vi "test1-LocalExternalStatusRegistration.vi"(8 "error in (no error)":errorcluster, 11 "TestCase in":refnum<class "testcase-CSMBroadcast.lvclass">) -> (0 "error out":errorcluster, 3 "TestCase out":refnum<class "testcase-CSMBroadcast.lvclass">)   [LabVIEW 2017, in "testcase-CSMBroadcast.lvclass"]
uses:
  testcase-CSMBroadcast.lvclass
  0b17d103-e67b-41be-a9eb-a2ee1311ff1f.vi
  5999693e-4f8a-4b34-ae87-f34dff5771be.vi
  de2dcf32-e0f3-4ce3-ae15-c78c2a65fbc0.vi
  52a2a10a-a04b-4bad-8df4-e1eb944f47cc.vi
  826f03dd-b4b5-4c6b-9085-8edf6da4f43b.vi
  src/user.lib/_NEVSTOP/Communicable State Machine(CSM)/AdvanceAPI/CSM - Revert Arguments-Safe String.vi
  src/user.lib/_NEVSTOP/Communicable State Machine(CSM)/AdvanceAPI/CSM - Make String Arguments Safe.vi
  src/user.lib/_NEVSTOP/Communicable State Machine(CSM)/AdvanceAPI/CSM - Break Down Multiple States String.vi
  src/user.lib/_NEVSTOP/Communicable State Machine(CSM)/AdvanceAPI/CSM - Keywords.vi
  src/user.lib/_NEVSTOP/Communicable State Machine(CSM)/_Polymophic/CSM - Replace Marks in Messages.vi
  src/user.lib/_NEVSTOP/Communicable State Machine(CSM)/AdvanceAPI/CSM - Get Module Attribute.vi
  src/user.lib/_NEVSTOP/Communicable State Machine(CSM)/_Shared/Trim Single-line Text.vi
  <vilib>/addons/_JKI Toolkits/VI Tester/TestCase.llb/TestCase.lvclass
  src/user.lib/_NEVSTOP/Communicable State Machine(CSM)/Communicable State Machine.lvlib
  CSM/CSM-Testcase.lvlib
  C:/Program Files (x86)/National Instruments/LabVIEW 2017/vi.lib/addons/_JKI Toolkits/VI Tester/TestCase.llb/TestCase.lvclass
panel:
  out "One-Shot Unregistrations":string
  out "One-Shot Registrations":string
  out "LoopCount 2":i32
  out "State History":string
  out "LoopCount":i32
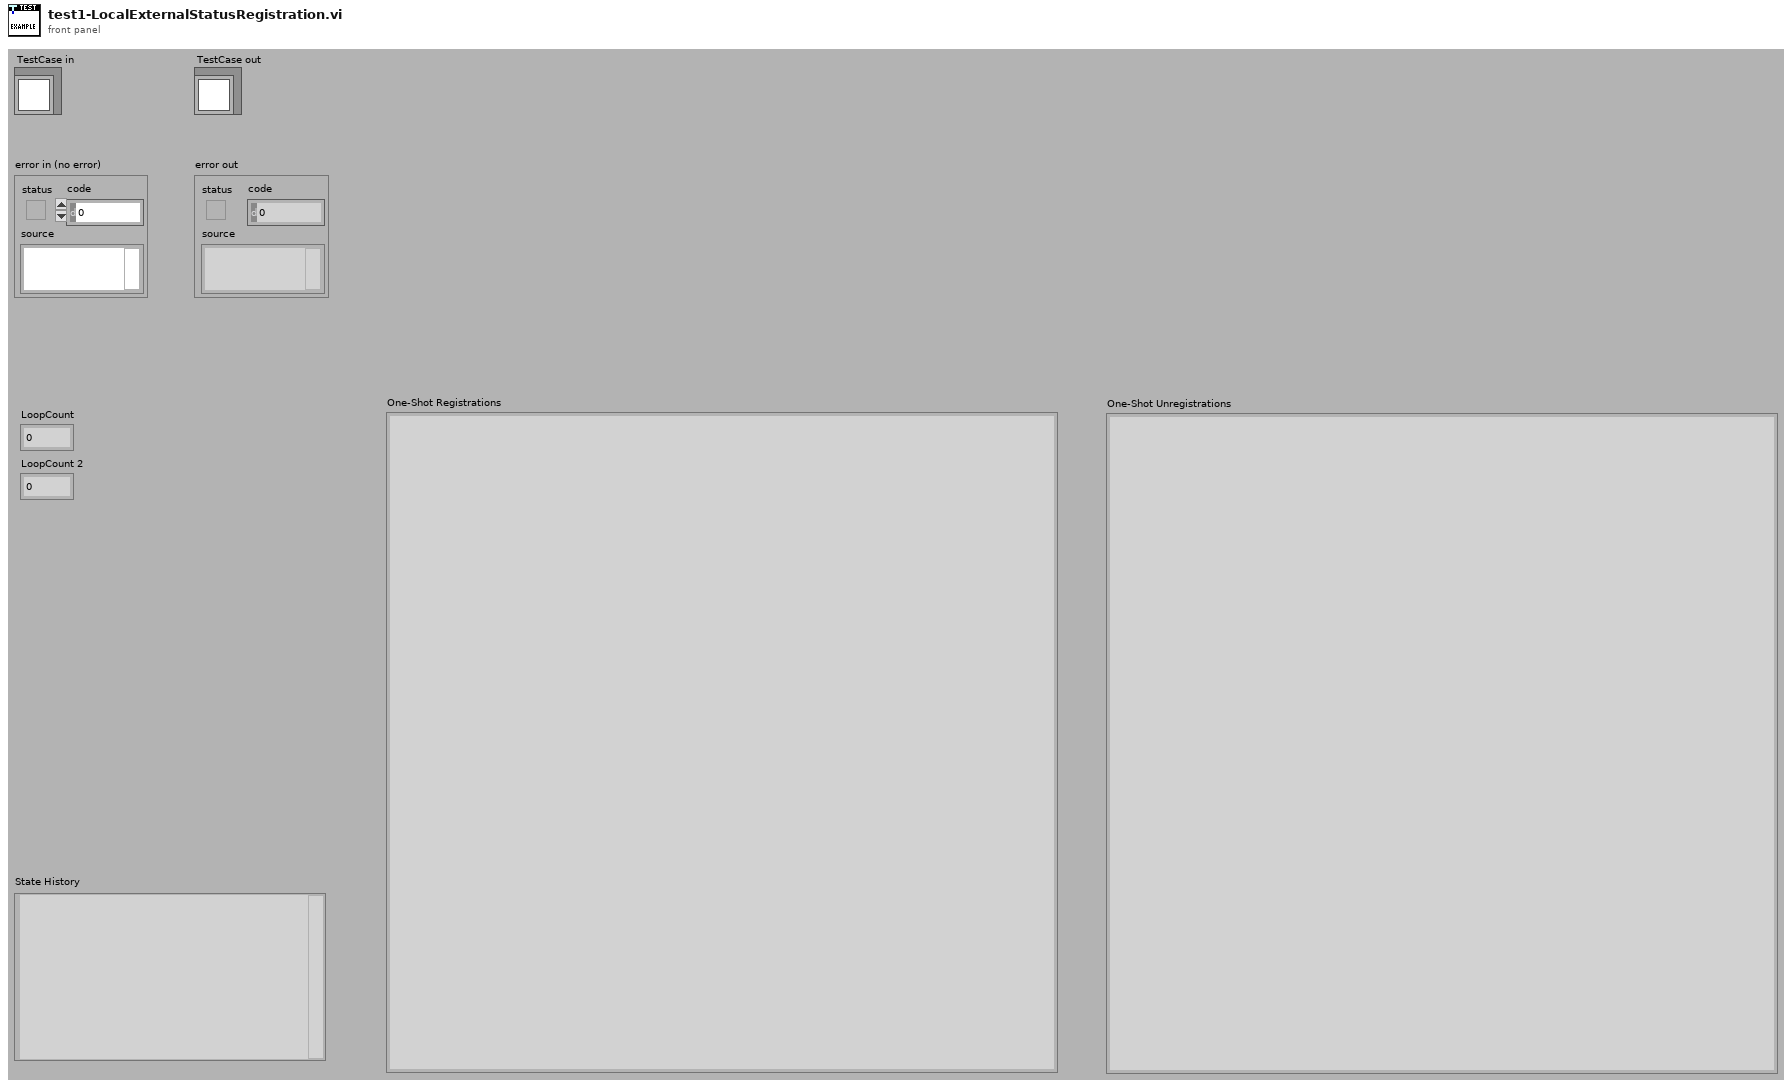
[diagram p1: front panel]
types:
  T1 = enum32{"Invalid", "Standard", "Closed", "Hidden", "Minimized", "Maximized"}
  T2 = enum32{"invalid app kind", "Development System", "Run Time System", "Student Edition", "Embedded LabVIEW", "Evaluation", "Custom"}
  T3 = typedef "Communicable State Machine.lvlib/_CSM_Response Source Message.ctl" = cluster{"‘State":string, "’Arguments":string, "’Error":errorcluster}
  T4 = cluster{"Current VI Reference":refnum<vi>, "Close Panel on Exit?":bool}
  T5 = cluster{"Core":cluster{"Current VI Reference":refnum<vi>, "Close Panel on Exit?":bool}, "Your Boolean data":bool, "Your string data":string}
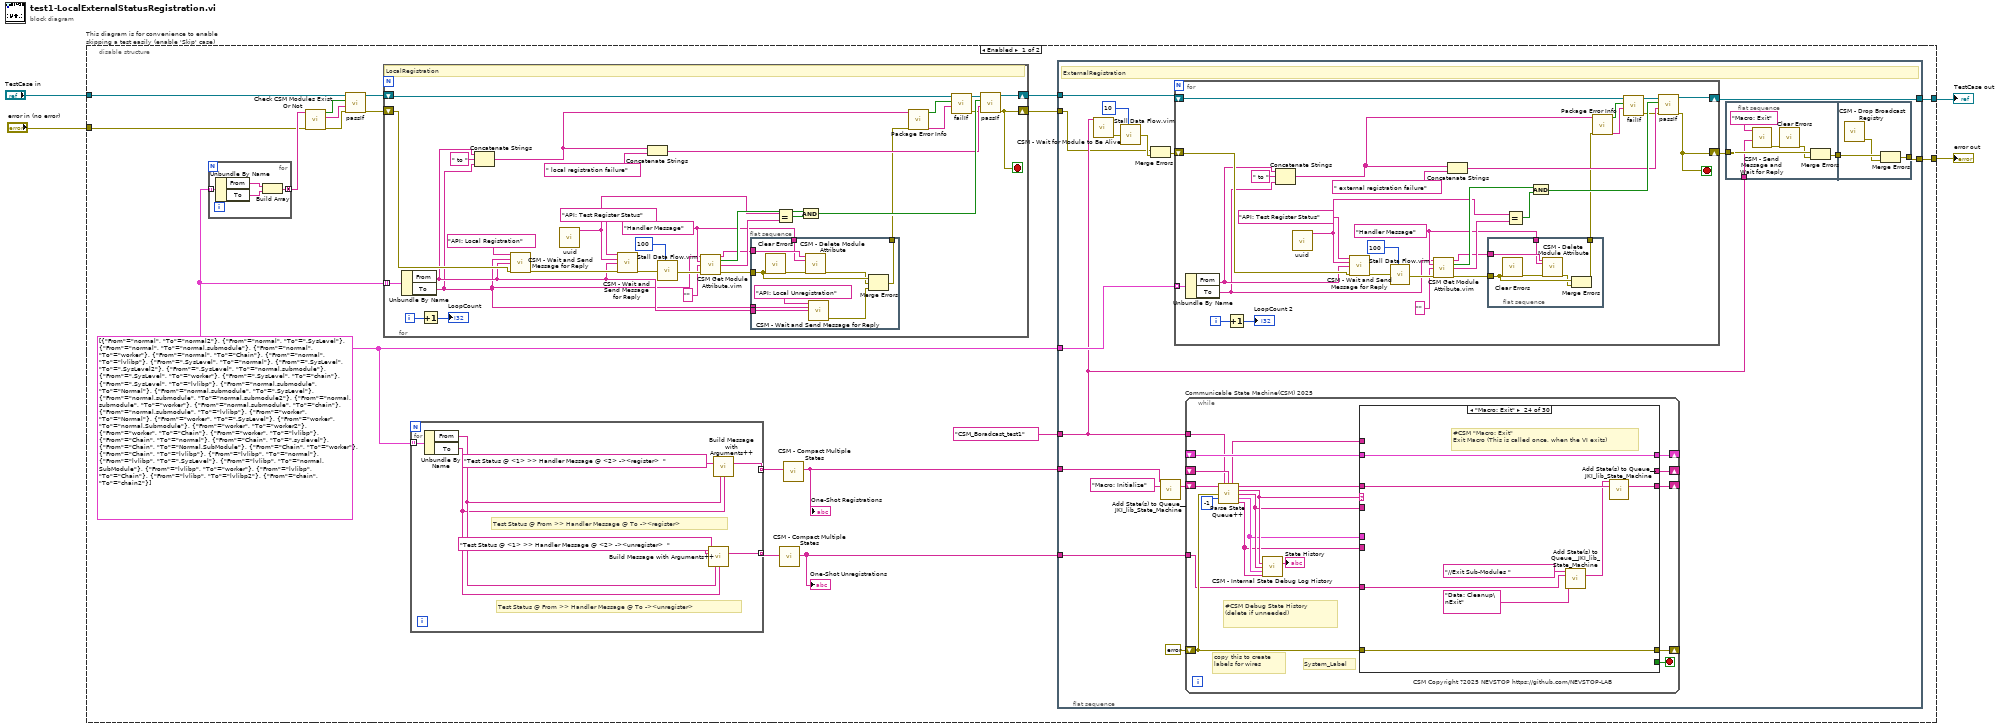
[diagram p0: block diagram]
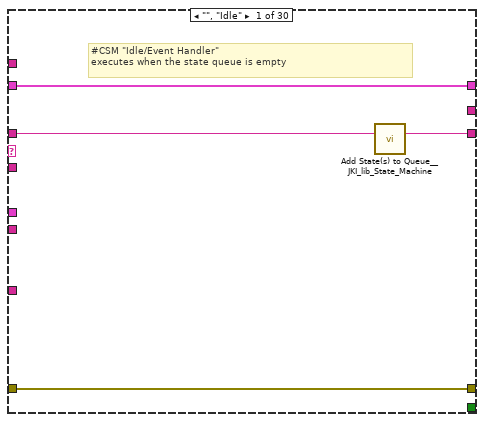
[diagram p2: hidden frame]
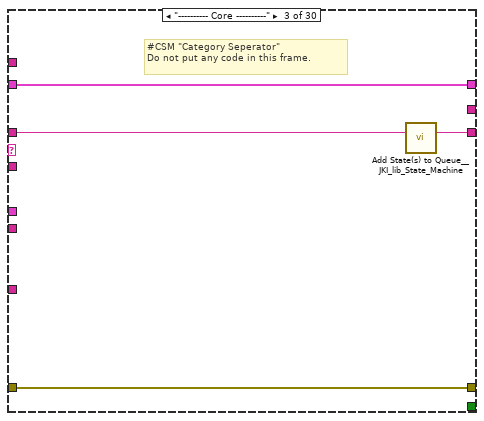
[diagram p4: hidden frame]
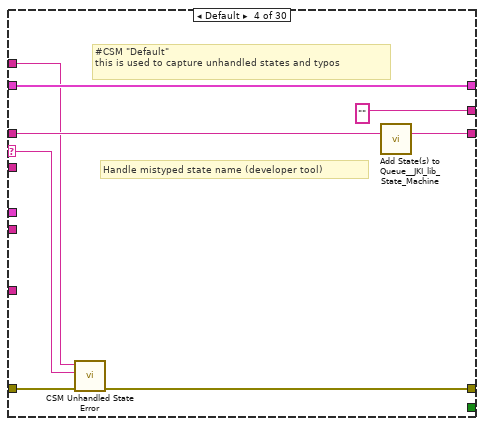
[diagram p5: hidden frame]
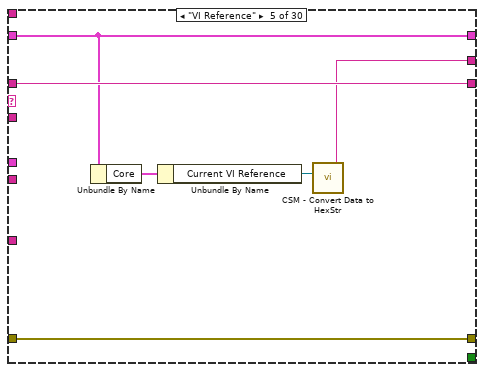
[diagram p6: hidden frame]
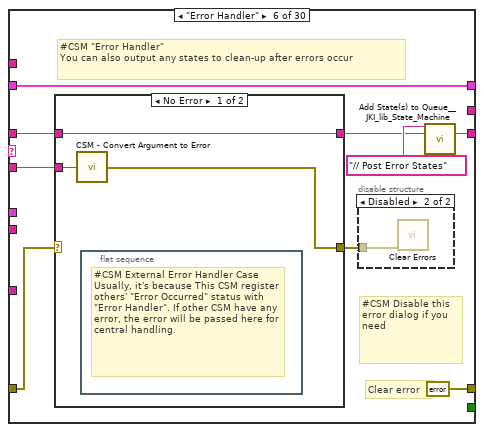
[diagram p7: hidden frame]
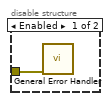
[diagram p8: hidden frame]
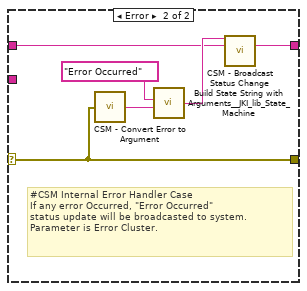
[diagram p9: hidden frame]
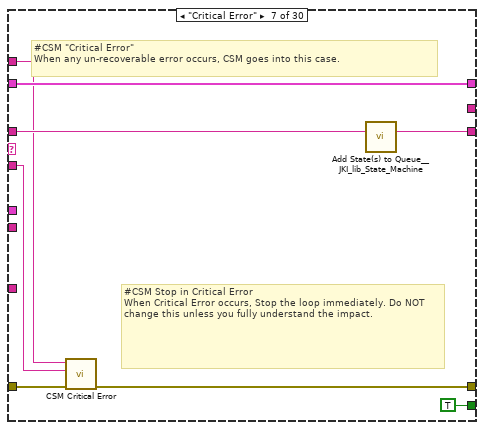
[diagram p10: hidden frame]
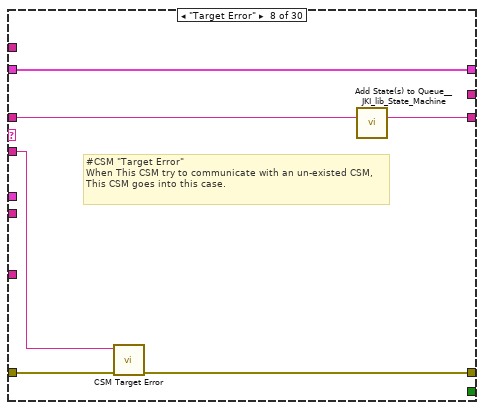
[diagram p11: hidden frame]
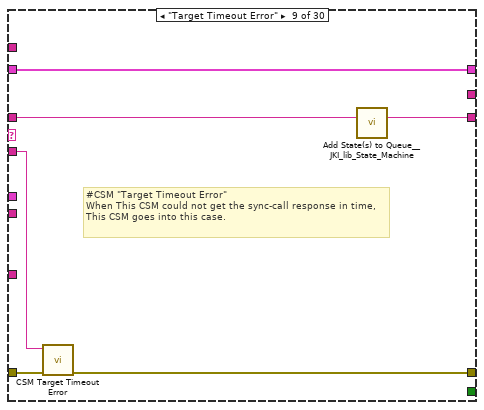
[diagram p12: hidden frame]
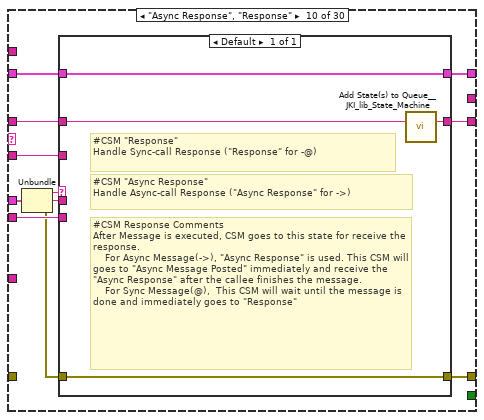
[diagram p13: hidden frame]
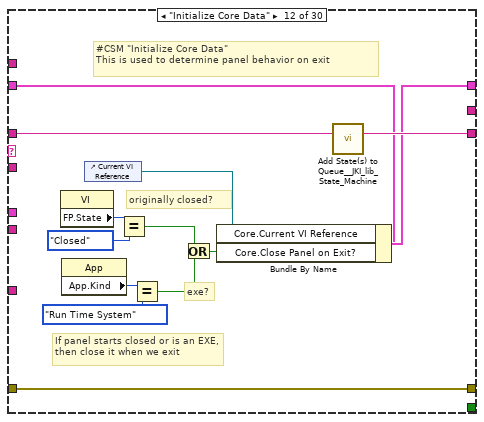
[diagram p15: hidden frame]
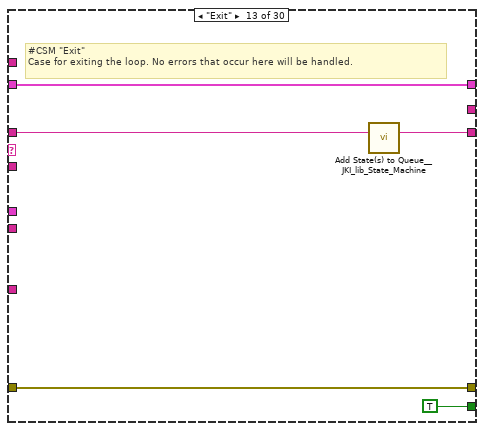
[diagram p16: hidden frame]
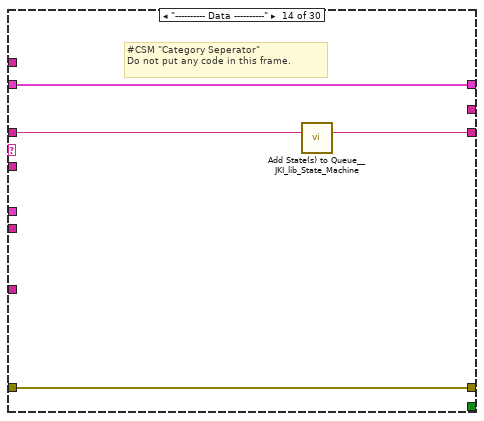
[diagram p17: hidden frame]
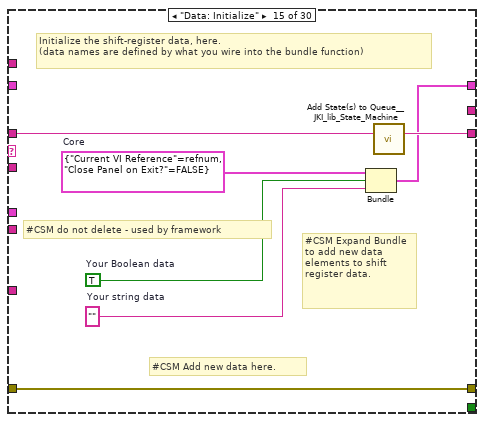
[diagram p18: hidden frame]
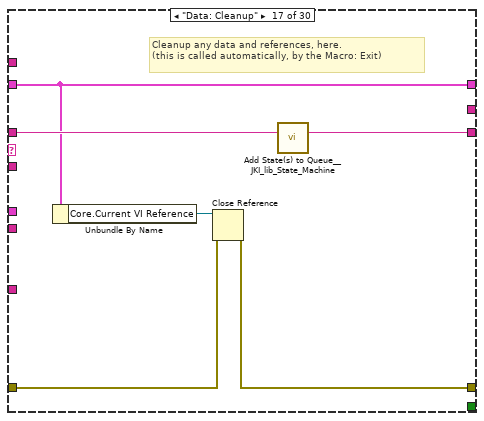
[diagram p20: hidden frame]
diagram:
  n1 = disable-structure "This diagram is for convenience to enable skipping a test easily (enable 'Skip' case)" shown="Enabled" {
    disable-tunnel: "TestCase in" -> [w10 w420]
    disable-tunnel: [w21 w418] -> w1
    disable-tunnel: [w15 w419] -> w3
    disable-tunnel: "error in (no error)" -> [w8 w417]
    frame Enabled {
      w7 = cluster{"From":string, "To":string}[] [{"From"="normal", "To"="normal2"}, {"From"="normal", "To"=".SysLevel"}, {"From"="normal", "To"="normal.submodule"}, {"From"="normal", "To"="worker"}, {"From"="normal", "To"="Chain"}, {"From"="normal", "To"="lvlibp"}, {"From"=".SysLevel", "To"="normal"}, {"From"=".SysLevel", "To"=".SysLevel2"}, {"From"=".SysLevel", "To"="normal.submodule"}, {"From"=".SysLevel", "To"="worker"}, {"From"=".SysLevel", "To"="chain"}, {"From"=".SysLevel", "To"="lvlibp"}, {"From"="normal.submodule", "To"="Normal"}, {"From"="normal.submodule", "To"=".SysLevel"}, {"From"="normal.submodule", "To"="normal.submodule2"}, {"From"="normal.submodule", "To"="worker"}, {"From"="normal.submodule", "To"="chain"}, {"From"="normal.submodule", "To"="lvlibp"}, {"From"="worker", "To"="Normal"}, {"From"="worker", "To"=".SysLevel"}, {"From"="worker", "To"="normal.Submodule"}, {"From"="worker", "To"="worker2"}, {"From"="worker", "To"="Chain"}, {"From"="worker", "To"="lvlibp"}, {"From"="Chain", "To"="normal"}, {"From"="Chain", "To"=".syslevel"}, {"From"="Chain", "To"="Normal.SubModule"}, {"From"="Chain", "To"="worker"}, {"From"="Chain", "To"="lvlibp"}, {"From"="lvlibp", "To"="normal"}, {"From"="lvlibp", "To"=".SysLevel"}, {"From"="lvlibp", "To"="normal.SubModule"}, {"From"="lvlibp", "To"="worker"}, {"From"="lvlibp", "To"="Chain"}, {"From"="lvlibp", "To"="lvlibp2"}, {"From"="chain", "To"="chain2"}]
      n2 = for {
        tunnel: w7 -> [w26] mode=indexing
        tunnel: [w23] -> w13 mode=concatenating
        n3 = Unbundle By Name(w26) -> ("From"=w25:string, "To"=w24:string)
        n4 = Build Array(w25, w24) -> (w23:string[])
      }
      n5 = call "Check CSM Modules Exist Or Not.vi"("error in"=w8, "CSM names in"=w13) -> ("error out"=w11:errorcluster, "Debug string"=w12:string, "All Modules Exist?"=w14:bool)  [unwired: 7 in]
      n6 = call-dynamic "passIf.vi"("error in (no error)"=w11, "message (\"\")"=w12, "pass"=w14, "TestCase in"=w10) -> ("error out"=w6:errorcluster, "TestCase out"=w9:refnum<class "testcase-CSMBroadcast.lvclass">)  [unwired: 6 in]
      n7 = for {
        shift-right: [w39] -> w20
        shift-left: w6 -> [w40]
        shift-right: [w46] -> w22
        shift-left: w9 -> [w31]
        tunnel: w7 -> [w57] mode=indexing
        i -> [w59]
        stop <- w39 stop-if-true
        w41 = "Handler Message" ("To")
        # "LocalRegistration"
        n8 = Unbundle By Name(w57) -> ("From"=w37:string, "To"=w36:string)
        n9 = Increment(x=w59) -> (x+1=→"LoopCount":i32)
        n10 = Concatenate Strings(w37, " to " ("string"), w36) -> (w27:string)
        n11 = call "CSM - Wait and Send Message for Reply.vi"("State"="API: Local Registration", "Arguments (\"\")"=w36, "Target Module"=w37, "Error In (No Error)"=w40) -> ("error out"=w54:errorcluster)  [unwired: 8 in, 3 out]
        n12 = call "uuid.vi"() -> ("UUID"=w48:string)  [unwired: 11 in]
        n13 = call "CSM - Wait and Send Message for Reply.vi"("State"="API: Test Register Status", "Arguments (\"\")"=w48, "Target Module"=w37, "Error In (No Error)"=w54) -> ("error out"=w53:errorcluster)  [unwired: 8 in, 3 out]
        n14 = Concatenate Strings(w27, " local registration failure" ("string")) -> (w34:string)
        n15 = call "Stall Data Flow.vim"("value in"=w53, "milliseconds to wait"=u32 100) -> ("value out"=w51:errorcluster)  [unwired: 1 out]
        n16 = call "CSM Get Module Attribute.vim"("CSM Name"=w36, "Attribute"=w41, "Default Value (Empty Variant)"="", "Error In"=w51) -> ("CSM Name (Dup)"=w42:string, "Found"=w50:bool, "Value"=w47:string, "error out"=w43:errorcluster)  [unwired: 7 in, 1 out]
        n17 = flat-sequence {
          tunnel: w43 -> [w63]
          tunnel: w42 -> [w68]
          tunnel: w41 -> [w67]
          tunnel: w36 -> [w65]
          tunnel: w37 -> [w64]
          tunnel: [w60] -> w28
          frame #0 {
            n18 = call <vilib>:"Clear Errors.vi"("error in (no error)"=w63) -> ("error out"=w69:errorcluster)  [unwired: 5 in, 1 out]
            n19 = call "CSM - Delete Module Attribute.vi"("CSM Name"=w68, "Attribute"=w67, "Error In"=w69) -> ("error out"=w62:errorcluster)  [unwired: 9 in, 3 out]
            n20 = call "CSM - Wait and Send Message for Reply.vi"("State"="API: Local Unregistration", "Arguments (\"\")"=w65, "Target Module"=w64) -> ("error out"=w61:errorcluster)  [unwired: 9 in, 3 out]
            n21 = Merge Errors(w63, w62, w61) -> (w60:errorcluster)
          }
        }
        n22 = Equal?(x=w48, y=w47) -> (x = y?=w45:bool)
        n23 = And(x=w50, y=w45) -> (x .and. y?=w44:bool)
        n24 = call "Package Error Info.vi"("error in"=w28, "String in"=w27) -> ("packed error info out"=w32:string, "error status"=w33:bool)  [unwired: 8 in]
        n25 = call-dynamic "failIf.vi"("message (\"\")"=w32, "fail"=w33, "TestCase in"=w31) -> ("error out"=w29:errorcluster, "TestCase out"=w30:refnum<class "testcase-CSMBroadcast.lvclass">)  [unwired: 7 in]
        n26 = call-dynamic "passIf.vi"("error in (no error)"=w29, "message (\"\")"=w34, "pass"=w44, "TestCase in"=w30) -> ("error out"=w39:errorcluster, "TestCase out"=w46:refnum<class "testcase-CSMBroadcast.lvclass">)  [unwired: 6 in]
      }
      n27 = for {
        tunnel: w7 -> [w75] mode=indexing
        tunnel: [w74] -> w19 mode=indexing
        tunnel: [w70] -> w17 mode=indexing
        # "Test Status @ From >> Handler Message @ To -><unregister>"
        # "Test Status @ From >> Handler Message @ To -><register>"
        n28 = Unbundle By Name(w75) -> ("From"=w72:string, "To"=w71:string)
        n29 = call-poly "Build Message with Arguments++.vi"("States With Replace Token"="Test Status @ <1> >> Handler Message @ <2> -><unregister>  " ("State"), "<1>"=w72, "<2>"=w71) -> ("States"=w70:string)  [unwired: 12 in]
        n30 = call-poly "Build Message with Arguments++.vi"("States With Replace Token"="Test Status @ <1> >> Handler Message @ <2> -><register>  " ("State"), "<1>"=w72, "<2>"=w71) -> ("States"=w74:string)  [unwired: 12 in]
      }
      n31 = call "CSM - Compact Multiple States.vi"("Multiple States"=w17) -> ("States"=w16:string)  [unwired: 9 in]
      "One-Shot Unregistrations" <- w16
      n32 = call "CSM - Compact Multiple States.vi"("Multiple States"=w19) -> ("States"=w18:string)  [unwired: 9 in]
      "One-Shot Registrations" <- w18
      n33 = flat-sequence {
        tunnel: w22 -> [w90]
        tunnel: [w89] -> w21
        tunnel: w20 -> [w77]
        tunnel: w7 -> [w88]
        tunnel: w18 -> [w87]
        tunnel: w16 -> [w84]
        tunnel: [w82] -> w15
        tunnel: "CSM_Boradcast_test1" ("Name (\"\" to Use UUID)") -> [w81]
        frame #0 {
          # "ExternalRegistration"
          n34 = call "CSM - Wait for Module to Be Alive.vi"("CSM Name"=w81) -> ("error out"=w80:errorcluster)  [unwired: 12 in, 2 out]
          n35 = call "Stall Data Flow.vim"("value in"=w80, "milliseconds to wait"=u32 10) -> ("value out"=w79:errorcluster)  [unwired: 1 out]
          n36 = Merge Errors(w77, w79) -> (w85:errorcluster)
          n37 = call <vilib>:"Add State(s) to Queue__JKI_lib_State_Machine.vi"("State(s) in Front (\"\")"=w87, "State(s) in (\"\")"="Macro: Initialize" ("Init State(\"Macro: Initialize\")")) -> ("States Out"=w91:string)  [unwired: 13 in]
          n38 = for {
            shift-right: [w115] -> w86
            shift-left: w85 -> [w116]
            shift-right: [w122] -> w89
            shift-left: w90 -> [w107]
            tunnel: w88 -> [w131] mode=indexing
            i -> [w133]
            stop <- w115 stop-if-true
            w117 = "Handler Message" ("To")
            n39 = Unbundle By Name(w131) -> ("From"=w112:string, "To"=w111:string)
            n40 = Increment(x=w133) -> (x+1=→"LoopCount 2":i32)
            n41 = Concatenate Strings(w112, " to " ("string"), w111) -> (w103:string)
            n42 = call "uuid.vi"() -> ("UUID"=w124:string)  [unwired: 11 in]
            n43 = call "CSM - Wait and Send Message for Reply.vi"("State"="API: Test Register Status", "Arguments (\"\")"=w124, "Target Module"=w112, "Error In (No Error)"=w116) -> ("error out"=w129:errorcluster)  [unwired: 8 in, 3 out]
            n44 = call "Stall Data Flow.vim"("value in"=w129, "milliseconds to wait"=u32 100) -> ("value out"=w127:errorcluster)  [unwired: 1 out]
            n45 = call "CSM Get Module Attribute.vim"("CSM Name"=w111, "Attribute"=w117, "Default Value (Empty Variant)"="", "Error In"=w127) -> ("CSM Name (Dup)"=w118:string, "Found"=w126:bool, "Value"=w123:string, "error out"=w119:errorcluster)  [unwired: 7 in, 1 out]
            n46 = Concatenate Strings(w103, " external registration failure" ("string")) -> (w110:string)
            n47 = flat-sequence {
              tunnel: w119 -> [w136]
              tunnel: w118 -> [w138]
              tunnel: w117 -> [w137]
              tunnel: [w134] -> w104
              frame #0 {
                n48 = call <vilib>:"Clear Errors.vi"("error in (no error)"=w136) -> ("error out"=w139:errorcluster)  [unwired: 5 in, 1 out]
                n49 = call "CSM - Delete Module Attribute.vi"("CSM Name"=w138, "Attribute"=w137, "Error In"=w139) -> ("error out"=w135:errorcluster)  [unwired: 9 in, 3 out]
                n50 = Merge Errors(w136, w135) -> (w134:errorcluster)
              }
            }
            n51 = Equal?(x=w124, y=w123) -> (x = y?=w121:bool)
            n52 = And(x=w126, y=w121) -> (x .and. y?=w120:bool)
            n53 = call "Package Error Info.vi"("error in"=w104, "String in"=w103) -> ("packed error info out"=w108:string, "error status"=w109:bool)  [unwired: 8 in]
            n54 = call-dynamic "failIf.vi"("message (\"\")"=w108, "fail"=w109, "TestCase in"=w107) -> ("error out"=w105:errorcluster, "TestCase out"=w106:refnum<class "testcase-CSMBroadcast.lvclass">)  [unwired: 7 in]
            n55 = call-dynamic "passIf.vi"("error in (no error)"=w105, "message (\"\")"=w110, "pass"=w120, "TestCase in"=w106) -> ("error out"=w115:errorcluster, "TestCase out"=w122:refnum<class "testcase-CSMBroadcast.lvclass">)  [unwired: 6 in]
          }
          n56 = while "Communicable State Machine(CSM) 2025" {
            shift-right: [w153] -> _
            shift-left: _ -> [w152]
            shift-right: [w156] -> _
            shift-left: errorcluster {"status"=FALSE, "code"=0, "source"=""} ("error out") -> [w151]
            shift-right: [w155] -> _
            shift-left: w91 -> [w157]
            shift-right: [w150] -> _
            shift-left: _ -> [w144]
            tunnel: w84 -> [w141]
            tunnel: w81 -> [w140]
            stop <- w154 stop-if-true
            # "#CSM Debug State History\n(delete if unneeded)"
            # "copy this to create labels for wires"
            # "System_Label"
            # "CSM Copyright ?2025 NEVSTOP https://github.com/NEVSTOP-LAB"
            n57 = call "Parse State Queue++.vi"("State Queue"=w157, "Name (\"\" to Use UUID)"=w140, "Response Arguments"=w144, "Previous Error"=w151, "Dequeue (1 ms)"=-1 ("Timeout")) -> ("Name Used"=w145:string, "Remaining States"=w158:string, "Current State"=w149:string, "Arguments"=w148:string, "Additional Information"=w147:T3, "Source CSM"=w146:string)  [unwired: 5 in]
            n58 = call "CSM - Internal State Debug Log History.vi"("State"=w149, "Arguments (\"\")"=w148, ">> Response Source Message >>"=w147, "Source (\"\")"=w146) -> ("Debug Log"=→"State History":string)  [unwired: 11 in]
            n59 = case shown="\"Macro: Exit\"" w149 {
              selector: w149 -> [_ _ _ w172 _ _ _ _ _ _ _ _ _ _ _ _ _ _ _ _ _ _ _ _ _ _ _ _ _ _]
              tunnel: w158 -> [w159 w164 w169 w176 w182 w188 w209 w215 w221 w229 w240 w254 w259 w263 w270 w272 w279 w283 w287 w293 w308 w377 w382 w390 w392 w396 w401 w408 w412 w416]
              tunnel: w148 -> [_ _ _ _ _ w187 w205 w214 w219 w228 _ _ _ _ _ _ _ _ _ w288 w302 _ _ _ _ _ w399 _ _ _]
              tunnel: w152 -> [w160 w163 w166 w174 w181 w191 w210 w216 w222 w231 w239 w247 w257 w260 _ w271 w274 w280 w285 w291 w304 w374 w379 w387 w391 w395 w400 w405 w409 w413]
              tunnel: [w161 w165 w167 w170 w183 errorcluster {"status"=FALSE, "code"=0, "source"=""} ("error out") w206 w212 w218 w234 w241 w251 w256 w261 w267 w273 w275 w281 w284 w289 w305 w375 w380 w388 w393 w397 w402 w406 w410 w414] -> w156
              tunnel: w151 -> [w161 w165 w167 w177 w183 w189 w211 w213 w220 _ w241 w251 w256 w261 w267 w273 w276 w281 w284 w290 w306 w375 w380 w388 w393 w397 w402 w406 w410 w414]
              tunnel: [w162 w164 w168 w175 w182 w184 w208 w217 w223 w230 w240 w253 w258 w262 w269 w272 w278 w282 w286 w292 w307 w376 w381 w389 w392 w396 w401 w407 w411 w415] -> w155
              tunnel: [_ _ _ _ _ _ TRUE _ _ _ _ _ TRUE _ _ _ _ _ _ _ _ _ _ _ _ _ _ _ _ _] -> w154
              tunnel: [w160 w163 w166 w174 w181 w191 w210 w216 w222 w232 w239 w252 w257 w260 w268 w271 w274 w280 w285 w291 w304 w374 w379 w387 w391 w395 w400 w405 w409 w413] -> w153
              tunnel: w146 -> [_ _ _ _ _ _ _ _ _ w226 _ _ _ _ _ _ _ _ _ _ _ _ _ _ _ _ _ _ _ _]
              tunnel: w147 -> [_ _ _ _ _ _ _ _ _ w233 _ _ _ _ _ _ _ _ _ _ _ _ _ _ _ _ _ _ _ _]
              tunnel: [_ _ _ "" w178 _ _ _ _ _ _ _ _ _ _ _ _ _ _ _ _ _ _ _ _ "API1 Response" w398 _ _ _] -> w150
              tunnel: w145 -> [_ _ _ w171 _ _ w204 _ _ _ _ _ _ _ _ _ _ _ _ _ _ _ _ _ _ _ _ _ _ _]
              tunnel: w141 -> [_ _ _ _ _ _ _ _ _ _ _ _ _ _ _ _ _ _ _ _ _ _ _ w383 _ _ _ _ _ _]
              frame "", "Idle" {
                # "#CSM \"Idle/Event Handler\"\nexecutes when the state queue is empty"
                n60 = call <vilib>:"Add State(s) to Queue__JKI_lib_State_Machine.vi"("State(s) in (\"\")"=w159) -> ("States Out"=w162:string)  [unwired: 14 in]
              }
              frame "CSM Documentation" {
                # "#CSM README FIRST\n\nCommunicable State Machine(CSM) is a LabVIEW application framework that builds upon JKI State Machine(JKISM). It follows the pattern of JKISM and extends the keywords to describe message communication between modules, including concepts such as Sync-Message, Async-Message, Subscription/Unsubscription of status - essential elements for creating reusable code modules. For more information, please visit the CSM wiki: https://nevstop-lab.github.io/CSM-Wiki/\n\nFor instructions on JKI State Machine, visit: http://jki.net/state-machine/\nFor information about CSM, visit: https://github.com/NEVSTOP-LAB"
                # "#CSM \"Documentation\"\nCase for holding CSM Documenation"
              }
              frame "---------- Core ----------" {
                # "#CSM \"Category Seperator\"\nDo not put any code in this frame."
                n61 = call <vilib>:"Add State(s) to Queue__JKI_lib_State_Machine.vi"("State(s) in (\"\")"=w169) -> ("States Out"=w168:string)  [unwired: 14 in]
              }
              frame Default {
                # "#CSM \"Default\"\nthis is used to capture unhandled states and typos"
                # "Handle mistyped state name (developer tool)"
                n62 = call "CSM Unhandled State Error.vi"("error in (no error)"=w177, "Undefined State"=w172, "CSM Name"=w171) -> ("error out"=w170:errorcluster)  [unwired: 8 in]
                n63 = call <vilib>:"Add State(s) to Queue__JKI_lib_State_Machine.vi"("State(s) in (\"\")"=w176) -> ("States Out"=w175:string)  [unwired: 14 in]
              }
              frame "VI Reference" {
                n64 = Unbundle By Name(w181) -> ("Core"=w180:T4)
                n65 = Unbundle By Name(w180) -> ("Current VI Reference"=w179:refnum<vi>)
                n66 = call "CSM - Convert Data to HexStr.vi"("Variant"=w179) -> ("HEX String (0-9,A-F)"=w178:string)  [unwired: 8 in]
              }
              frame "Error Handler" {
                # "#CSM Disable this error dialog if you need"
                # "#CSM \"Error Handler\"\nYou can also output any states to clean-up after errors occur"
                # "Clear error"
                n67 = case shown="No Error" w189 {
                  selector: w189 -> [_ w198]
                  tunnel: [w197 w200] -> w185
                  tunnel: w188 -> [w197 w199]
                  tunnel: w187 -> [w196 _]
                  tunnel: [w195 w198] -> w190
                  frame No Error {
                    n68 = call "CSM - Convert Argument to Error.vi"("Argument"=w196) -> ("Error"=w195:errorcluster)  [unwired: 4 in]
                    n69 = flat-sequence {
                      frame #0 {
                        # "#CSM External Error Handler Case\nUsually, it's because This CSM register others' \"Error Occurred\" status with \"Error Handler\". If other CSM have any error, the error will be passed here for central handling."
                      }
                    }
                  }
                  frame Error {
                    # "#CSM Internal Error Handler Case \nIf any error Occurred, \"Error Occurred\" \nstatus update will be broadcasted to system.\nParameter is Error Cluster."
                    n70 = call "CSM - Convert Error to Argument.vi"("Error"=w198) -> ("Argument"=w202:string)  [unwired: 4 in]
                    n71 = call <vilib>:"Build State String with Arguments__JKI_lib_State_Machine.vi"("Arguments (\"\")"=w202, "State"="Error Occurred" ("Status with Arguments")) -> ("State with Arguments"=w201:string)  [unwired: 4 in]
                    n72 = call "CSM - Broadcast Status Change.vi"("Status With Arguments"=w201, "State Queue"=w199) -> ("Remaining States"=w200:string)  [unwired: 13 in]
                  }
                }
                n73 = disable-structure shown="Disabled" {
                  disable-tunnel: w190 -> [w193 w194]
                  frame Enabled {
                    n74 = call <vilib>:"General Error Handler.vi"("error in (no error)"=w193) -> ()  [unwired: 10 in, 5 out]
                  }
                  frame Disabled {
                    n75 = call <vilib>:"Clear Errors.vi"("error in (no error)"=w194) -> ()  [unwired: 5 in, 2 out]
                  }
                }
                n76 = call <vilib>:"Add State(s) to Queue__JKI_lib_State_Machine.vi"("State(s) in Front (\"\")"="// Post Error States", "State(s) in (\"\")"=w185) -> ("States Out"=w184:string)  [unwired: 13 in]
              }
              frame "Critical Error" {
                # "#CSM Stop in Critical Error\nWhen Critical Error occurs, Stop the loop immediately. Do NOT change this unless you fully understand the impact."
                # "#CSM \"Critical Error\"\nWhen any un-recoverable error occurs, CSM goes into this case."
                n77 = call "CSM Critical Error.vi"("error in (no error)"=w211, "Arugments (As Reason)"=w205, "CSM Name"=w204) -> ("error out"=w206:errorcluster)  [unwired: 8 in]
                n78 = call <vilib>:"Add State(s) to Queue__JKI_lib_State_Machine.vi"("State(s) in (\"\")"=w209) -> ("States Out"=w208:string)  [unwired: 14 in]
              }
              frame "Target Error" {
                # "#CSM \"Target Error\"\nWhen This CSM try to communicate with an un-existed CSM, This CSM goes into this case."
                n79 = call "CSM Target Error.vi"("error in (no error)"=w213, "Arguments (As CSM Name)"=w214) -> ("error out"=w212:errorcluster)  [unwired: 9 in]
                n80 = call <vilib>:"Add State(s) to Queue__JKI_lib_State_Machine.vi"("State(s) in (\"\")"=w215) -> ("States Out"=w217:string)  [unwired: 14 in]
              }
              frame "Target Timeout Error" {
                # "#CSM \"Target Timeout Error\"\nWhen This CSM could not get the sync-call response in time, This CSM goes into this case."
                n81 = call "CSM Target Timeout Error.vi"("error in (no error)"=w220, "Arguments (As CSM Name)"=w219) -> ("error out"=w218:errorcluster)  [unwired: 9 in]
                n82 = call <vilib>:"Add State(s) to Queue__JKI_lib_State_Machine.vi"("State(s) in (\"\")"=w221) -> ("States Out"=w223:string)  [unwired: 14 in]
              }
              frame "Async Response", "Response" {
                n83 = Unbundle(w233) -> ("‘State"=w227:string, "’Arguments"=w225:string, "’Error"=w224:errorcluster)
                n84 = case shown="Default" w227 {
                  tunnel: [w238] -> w234
                  tunnel: w224 -> [w238]
                  tunnel: [w237] -> w232
                  tunnel: w231 -> [w237]
                  tunnel: [w235] -> w230
                  tunnel: w229 -> [w236]
                  tunnel: w228 -> [_]
                  tunnel: w226 -> [_]
                  tunnel: w225 -> [_]
                  frame Default {
                    # "#CSM Response Comments\nAfter Message is executed, CSM goes to this state for receive the response.\n    For Async Message(->), \"Async Response\" is used. This CSM will goes to \"Async Message Posted\" immediately and receive the \"Async Response\" after the callee finishes the message.\n    For Sync Message(@),  This CSM will wait until the message is done and immediately goes to \"Response\""
                    # "#CSM \"Async Response\"\nHandle Async-call Response (\"Async Response\" for ->)"
                    # "#CSM \"Response\"\nHandle Sync-call Response (\"Response\" for -@)"
                    n85 = call <vilib>:"Add State(s) to Queue__JKI_lib_State_Machine.vi"("State(s) in (\"\")"=w236) -> ("States Out"=w235:string)  [unwired: 14 in]
                  }
                }
              }
              frame "Async Message Posted" {
                # "#CSM \"Async Message Posted\"\nAfter Async Message is posted (-> or ->| ), CSM goes to this state for post-action.\nYou can use Argument - State to tell which Async Message is called."
              }
              frame "Initialize Core Data" {
                # "#CSM \"Initialize Core Data\"\nThis is used to determine panel behavior on exit"
                # "originally closed?"
                # "exe?"
                # "If panel starts closed or is an EXE, then close it when we exit"
                n86 = property class="VI"() -> ("FP.State"=w244:T1)  [unwired: 2 in, 2 out]
                n87 = property class="App"() -> ("App.Kind"=w250:T2)  [unwired: 2 in, 2 out]
                n88 = control-ref of="Current VI Reference"() -> (w245:refnum<vi>)
                n89 = Equal?(x=w244, y=T1."Closed" ("Front Panel Window:State")) -> (x = y?=w242:bool)
                n90 = Equal?(x=w250, y=T2."Run Time System" ("Application:Kind")) -> (x = y?=w248:bool)
                n91 = Or(x=w242, y=w248) -> (x .or. y?=w246:bool)
                n92 = Bundle By Name(cluster=w247, "Core.Current VI Reference"=w245, "Core.Close Panel on Exit?"=w246) -> (w252:T5)
                n93 = call <vilib>:"Add State(s) to Queue__JKI_lib_State_Machine.vi"("State(s) in (\"\")"=w254) -> ("States Out"=w253:string)  [unwired: 14 in]
              }
              frame "Exit" {
                # "#CSM \"Exit\"\nCase for exiting the loop. No errors that occur here will be handled."
                n94 = call <vilib>:"Add State(s) to Queue__JKI_lib_State_Machine.vi"("State(s) in (\"\")"=w259) -> ("States Out"=w258:string)  [unwired: 14 in]
              }
              frame "---------- Data ----------" {
                # "#CSM \"Category Seperator\"\nDo not put any code in this frame."
                n95 = call <vilib>:"Add State(s) to Queue__JKI_lib_State_Machine.vi"("State(s) in (\"\")"=w263) -> ("States Out"=w262:string)  [unwired: 14 in]
              }
              frame "Data: Initialize" {
                w264 = T4 {"Current VI Reference"=refnum, "Close Panel on Exit?"=FALSE}  # Core
                w266 = TRUE  # Your Boolean data
                w265 = ""  # Your string data
                # "#CSM do not delete - used by framework"
                # "#CSM Expand Bundle to add new data elements to shift register data."
                # "#CSM Add new data here."
                # "Initialize the shift-register data, here.\n(data names are defined by what you wire into the bundle function)"
                n96 = Bundle("Core"=w264, "Your Boolean data"=w266, "Your string data"=w265) -> (w268:T5)  [unwired: 1 in]
                n97 = call <vilib>:"Add State(s) to Queue__JKI_lib_State_Machine.vi"("State(s) in (\"\")"=w270) -> ("States Out"=w269:string)  [unwired: 14 in]
              }
              frame "Data: Update Indicators" {
              }
              frame "Data: Cleanup" {
                # "Cleanup any data and references, here.\n(this is called automatically, by the Macro: Exit)"
                n98 = Unbundle By Name(w274) -> ("Core.Current VI Reference"=w277:refnum<vi>)
                n99 = Close Reference(reference=w277, error in (no error)=w276) -> (error out=w275:errorcluster)
                n100 = call <vilib>:"Add State(s) to Queue__JKI_lib_State_Machine.vi"("State(s) in (\"\")"=w279) -> ("States Out"=w278:string)  [unwired: 14 in]
              }
              frame "---------- UI ----------" {
                # "#CSM \"Category Seperator\"\nDo not put any code in this frame."
                n101 = call <vilib>:"Add State(s) to Queue__JKI_lib_State_Machine.vi"("State(s) in (\"\")"=w283) -> ("States Out"=w282:string)  [unwired: 14 in]
              }
              frame "UI: Initialize" {
                # "#CSM \"UI: Initialize\"\nInitialize the User Interface, here.\n(this is called automatically, by the Macro: Init)"
                n102 = call <vilib>:"Add State(s) to Queue__JKI_lib_State_Machine.vi"("State(s) in (\"\")"=w287) -> ("States Out"=w286:string)  [unwired: 14 in]
              }
              frame "UI: Cursor Set" {
                # "#CSM \"UI: Cursor Set\"\nSet and Unset Cursor Busy.\n(Usage: \"UI: Cursor Set >> Busy|Idle\")"
                # "Argument"
                n103 = disable-structure shown="TARGET_TYPE!=Windows" {
                  disable-tunnel: w290 -> [w296 w301]
                  disable-tunnel: [w295 w301] -> w289
                  disable-tunnel: w288 -> [w294 _]
                  frame condition #0 (active) {
                    n104 = case shown="\"Idle\", Default" w294 {
                      tunnel: w296 -> [w298 w300]
                      tunnel: [w297 w299] -> w295
                      frame "Idle", Default {
                        n105 = call <vilib>:"Unset Busy.vi"("error in (no error)"=w298) -> ("error out"=w297:errorcluster)  [unwired: 10 in]
                      }
                      frame "Busy" {
                        n106 = call <vilib>:"Set Busy.vi"("error in (no error)"=w300) -> ("error out"=w299:errorcluster)  [unwired: 9 in, 1 out]
                      }
                    }
                  }
                  frame condition #1 {
                  }
                }
                n107 = call <vilib>:"Add State(s) to Queue__JKI_lib_State_Machine.vi"("State(s) in (\"\")"=w293) -> ("States Out"=w292:string)  [unwired: 14 in]
              }
              frame "UI: Front Panel State" {
                # "#CSM \"UI: Front Panel State\"\nSet Front Panel Open or Closed\n(Usage: \"UI: Front Panel State >> Open|Close\")"
                # "Argument"
                n108 = Unbundle By Name(w304) -> ("Core.Current VI Reference"=w303:refnum<vi>)
                n109 = call <vilib>:"Add State(s) to Queue__JKI_lib_State_Machine.vi"("State(s) in (\"\")"=w308) -> ("States Out"=w307:string)  [unwired: 14 in]
                n110 = case shown="\"Close\", \"Closed\"" w302 {
                  tunnel: w306 -> [w314 w329 w340 w353 w366]
                  tunnel: [w316 w330 w342 w355 w368] -> w305
                  tunnel: w303 -> [w315 w327 w341 w354 w367]
                  frame "Open", "Standard", Default {
                    w309 = T1."Standard" ("State")
                    n111 = property class="VI"(reference=w315, error in=w314) -> (reference out=w312:refnum<vi>, error out=w313:errorcluster, "FP.State"=w311:T1)
                    n112 = Not Equal?(x=w311, y=w309) -> (x != y?=w310:bool)
                    n113 = case shown="True" w310 {
                      tunnel: [w320 w322] -> w316
                      tunnel: w313 -> [w319 w322]
                      tunnel: w312 -> [w318 _]
                      tunnel: w309 -> [w317 _]
                      frame True {
                        n114 = invoke class="VI" method="FP.Open"(reference=w318, error in=w319, "Activate"=TRUE, "State"=w317) -> (error out=w320:errorcluster)  [unwired: 1 in, 4 out]
                      }
                      frame False {
                      }
                    }
                  }
                  frame "Close", "Closed" {
                    n115 = property class="VI"(reference=w327, error in=w329) -> (reference out=w326:refnum<vi>, error out=w328:errorcluster, "FP.State"=w324:T1)
                    n116 = Not Equal?(x=w324, y=T1."Closed" ("Front Panel Window:State")) -> (x != y?=w323:bool)
                    n117 = case shown="False" w323 {
                      tunnel: [w331 w334] -> w330
                      tunnel: w328 -> [w331 w333]
                      tunnel: w326 -> [_ w332]
                      frame False {
                      }
                      frame True {
                        n118 = invoke class="VI" method="FP.Close"(reference=w332, error in=w333) -> (error out=w334:errorcluster)  [unwired: 1 in, 2 out]
                      }
                    }
                  }
                  frame "Hidden", "Hide" {
                    w335 = T1."Hidden" ("State")
                    n119 = property class="VI"(reference=w341, error in=w340) -> (reference out=w338:refnum<vi>, error out=w339:errorcluster, "FP.State"=w337:T1)
                    n120 = Not Equal?(x=w337, y=w335) -> (x != y?=w336:bool)
                    n121 = case shown="True" w336 {
                      tunnel: [w346 w347] -> w342
                      tunnel: w339 -> [w345 w347]
                      tunnel: w338 -> [w344 _]
                      tunnel: w335 -> [w343 _]
                      frame True {
                        n122 = invoke class="VI" method="FP.Open"(reference=w344, error in=w345, "State"=w343) -> (error out=w346:errorcluster)  [unwired: 2 in, 4 out]
                      }
                      frame False {
                      }
                    }
                  }
                  frame "Minimize", "Minimized" {
                    w348 = T1."Minimized" ("State")
                    n123 = property class="VI"(reference=w354, error in=w353) -> (reference out=w351:refnum<vi>, error out=w352:errorcluster, "FP.State"=w350:T1)
                    n124 = Not Equal?(x=w350, y=w348) -> (x != y?=w349:bool)
                    n125 = case shown="True" w349 {
                      tunnel: [w359 w360] -> w355
                      tunnel: w352 -> [w358 w360]
                      tunnel: w351 -> [w357 _]
                      tunnel: w348 -> [w356 _]
                      frame True {
                        n126 = invoke class="VI" method="FP.Open"(reference=w357, error in=w358, "State"=w356) -> (error out=w359:errorcluster)  [unwired: 2 in, 4 out]
                      }
                      frame False {
                      }
                    }
                  }
                  frame "Maximize", "Maximized" {
                    w361 = T1."Maximized" ("State")
                    n127 = property class="VI"(reference=w367, error in=w366) -> (reference out=w364:refnum<vi>, error out=w365:errorcluster, "FP.State"=w363:T1)
                    n128 = Not Equal?(x=w363, y=w361) -> (x != y?=w362:bool)
                    n129 = case shown="True" w362 {
                      tunnel: [w372 w373] -> w368
                      tunnel: w365 -> [w371 w373]
                      tunnel: w364 -> [w370 _]
                      tunnel: w361 -> [w369 _]
                      frame True {
                        n130 = invoke class="VI" method="FP.Open"(reference=w370, error in=w371, "State"=w369) -> (error out=w372:errorcluster)  [unwired: 2 in, 4 out]
                      }
                      frame False {
                      }
                    }
                  }
                }
              }
              frame "---------- Macro ----------" {
                # "#CSM \"Category Seperator\"\nDo not put any code in this frame."
                n131 = call <vilib>:"Add State(s) to Queue__JKI_lib_State_Machine.vi"("State(s) in (\"\")"=w377) -> ("States Out"=w376:string)  [unwired: 14 in]
              }
              frame "Macro: Initialize" {
                # "#CSM \"Macro: Initialize\"\nInitialization Macro (This is called once, when the VI starts)"
                n132 = call <vilib>:"Add State(s) to Queue__JKI_lib_State_Machine.vi"("State(s) in Front (\"\")"="Data: Initialize\nInitialize Core Data\nData: Update Indicators", "State(s) in (\"\")"=w382) -> ("States Out"=w381:string)  [unwired: 13 in]
              }
              frame "Macro: Exit" {
                # "#CSM \"Macro: Exit\"\nExit Macro (This is called once, when the VI exits)"
                n133 = call <vilib>:"Add State(s) to Queue__JKI_lib_State_Machine.vi"("State(s) in Front (\"\")"="//Exit Sub-Modules ", "State(s) in (\"\")"=w383, "State(s) at Back (\"\")"="Data: Cleanup\nExit") -> ("States Out"=w385:string)  [unwired: 12 in]
                n134 = call <vilib>:"Add State(s) to Queue__JKI_lib_State_Machine.vi"("State(s) in Front (\"\")"=w385, "State(s) in (\"\")"=w390) -> ("States Out"=w389:string)  [unwired: 13 in]
              }
              frame "---------- API ----------" {
                # "#CSM \"Category Seperator\"\nDo not put any code in this frame."
              }
              frame "API: API1" {
                # "#CSM API Example\nCopy/Rename this case for your own API"
                # "#CSM Response\nConnect this to return the response of your API"
                # "#CSM >> Msg/Rep's CSM >>\nIf you need to tell who triggered this state , use this string. If it's this case itself, this string is \"\"."
                # "#CSM >> Arguments >>\nDeal with the parameter if any"
              }
              frame "API: API2" {
                # "#CSM API Example\nCopy/Rename this case for your own API"
                # "unpack Hex String  to Variant\nif complex parameter is needed."
                n135 = call "CSM - Convert HexStr to Data.vi"("HEX String"=w399) -> ()  [unwired: 7 in, 2 out]
                n136 = disable-structure shown="Disabled" {
                  disable-tunnel: [w403 "API2 Response"] -> w398
                  frame Disabled {
                    # "pack variant to hexstr \nif complex response is needed."
                    # "complex Response"
                    n137 = call "CSM - Convert Data to HexStr.vi"() -> ("HEX String (0-9,A-F)"=w403:string)  [unwired: 9 in]
                  }
                  frame Enabled {
                  }
                }
              }
              frame "---------- Action ----------" {
                # "#CSM \"Category Seperator\"\nDo not put any code in this frame."
                n138 = call <vilib>:"Add State(s) to Queue__JKI_lib_State_Machine.vi"("State(s) in (\"\")"=w408) -> ("States Out"=w407:string)  [unwired: 14 in]
              }
              frame "Action: action1" {
                # "#CSM \"Internal State\"\nThis category is used for holding internal states"
                n139 = call <vilib>:"Add State(s) to Queue__JKI_lib_State_Machine.vi"("State(s) in (\"\")"=w412) -> ("States Out"=w411:string)  [unwired: 14 in]
              }
              frame "Action: action2" {
                # "#CSM \"Internal State\"\nThis category is used for holding internal states"
                n140 = call <vilib>:"Add State(s) to Queue__JKI_lib_State_Machine.vi"("State(s) in (\"\")"=w416) -> ("States Out"=w415:string)  [unwired: 14 in]
              }
            }
          }
          n141 = flat-sequence {
            tunnel: w86 -> [w98]
            tunnel: [w97] -> w83
            tunnel: w81 -> [w96]
            tunnel: w83 -> [w102]
            tunnel: [w101] -> w82
            frame #0 {
              n142 = call "CSM - Send Message and Wait for Reply.vi"("Target Module"=w96, "State"="Macro: Exit") -> ("error out"=w95:errorcluster)  [unwired: 7 in, 2 out]
              n143 = call <vilib>:"Clear Errors.vi"("error in (no error)"=w95) -> ("error out"=w94:errorcluster)  [unwired: 5 in, 1 out]
              n144 = Merge Errors(w98, w94) -> (w97:errorcluster)
            }
            frame #1 {
              n145 = call "CSM - Drop Broadcast Registry.vi"() -> ("error out"=w100:errorcluster)  [unwired: 15 in]
              n146 = Merge Errors(w102, w100) -> (w101:errorcluster)
            }
          }
        }
      }
    }
    frame Disabled {
      # "skip test result while test is under development"
      n147 = call <vilib>:"skip.vi"("error in (no error)"=w417, "TestCase in"=w420) -> ("error out"=w419:errorcluster, "TestCase out"=w418:refnum<class "testcase-CSMBroadcast.lvclass">)  [unwired: 8 in]
    }
  }
  "error out" <- w3
  "TestCase out" <- w1
